vi "Helper SubVI - Simulate ECG Signal.vi"() -> (3 "Data":dynamicdata(graph))   [LabVIEW 2023]
doc: "Simulates an ECG signal."
uses:
  Instance           3 30Saved   subSimulate ECG Signal .vi
  <vilib>/measure/NI_MABase.lvlib
  <vilib>/Analysis/NI_AALBase.lvlib
panel:
  in  "Simulate Acquisition Timing?":bool=TRUE
  in  "Amplitude":dbl=1.0 format="%0.2f"
  in  "Isoelectric Voltage":dbl format="%0.2f"
  out "error out":errorcluster
  in  "QRS-T Delay (ms)":dbl(slide)=22.0 scale=0.0..40.0
  in  "P-QRS Delay (ms)":dbl(slide)=22.0 scale=0.0..40.0
  in  "60 Hz Noise\nAmplitude":dbl(knob) scale=0.0..1.0
  in  "White Noise \nAmplitude":dbl(knob) scale=0.0..1.0
  in  "error in (no error)":errorcluster
  in  "Number of Samples":i32=500
  in  "BPM":dbl(knob)=80.0 scale=40.0..140.0
  in  "Signal Type":T1(ring)=enum."Normal (random)"
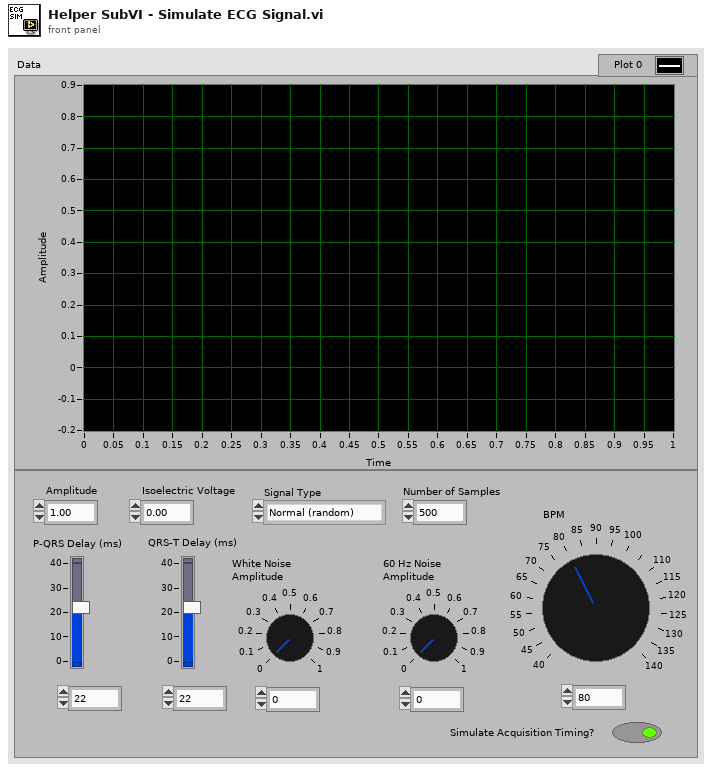
[diagram p1: front panel]
types:
  T1 = enum16{"Normal (regular)", "Normal (random)", "Hyperkalemia", "Atrial Tachycardia"}
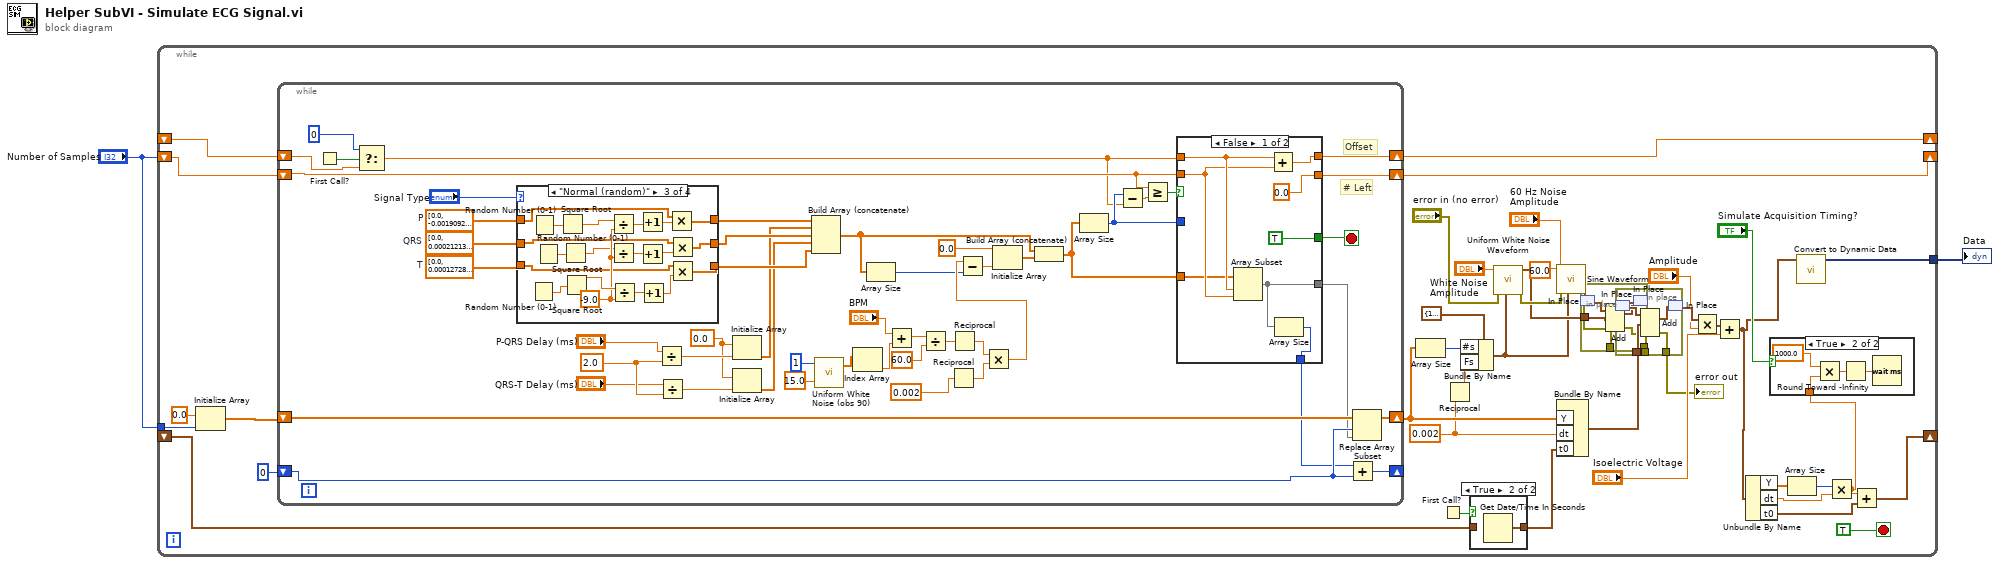
[diagram p0: block diagram]
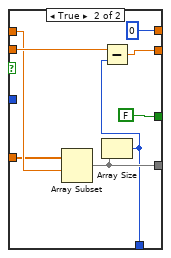
[diagram p4: hidden frame]
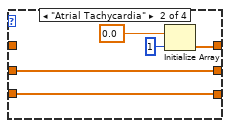
[diagram p6: hidden frame]
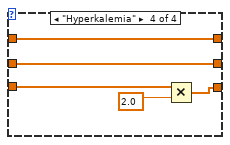
[diagram p7: hidden frame]
diagram:
  n1 = while {
    shift-right: [w6] -> _
    shift-left: _ -> [w36]
    shift-right: [w45] -> _
    shift-left: _ -> [w43]
    shift-right: [w44] -> _
    shift-left: "Number of Samples" -> [w42]
    tunnel: "Number of Samples" -> [w35]
    tunnel: [w3] -> w1
    stop <- TRUE stop-if-true
    w22 = 0.002 ("dt")
    n2 = Initialize Array(0.0 ("element"), w35) -> (w39:dbl[])
    n3 = while {
      shift-right: [w83] -> w45
      shift-left: w43 -> [w89]
      shift-right: [w82] -> w44
      shift-left: w42 -> [w86]
      shift-right: [w79] -> w26
      shift-left: w39 -> [w78]
      shift-right: [w77] -> _
      shift-left: 0 -> [w76]
      stop <- w87 stop-if-true
      w70 = dbl[] [0.0, 0.00012728044123886295, 0.0033092914722104368, 0.004963937208315655, 0.008909630886720407, 0.010691557064064489, 0.01463725074246924, 0.01641917691981332, 0.019601187950784894, 0.019983029274501487, 0.02189223589308443, 0.02609249045396691, 0.029529062367416203, 0.032965634280865505, 0.03703860840050912, 0.03945693678404752, 0.03971149766652524, 0.04174798472634705, 0.04645736105218498, 0.049130250318201105, 0.04951209164191769, 0.05167585914297836, 0.05434874840899448, 0.054730589732711075, 0.057403478998727185, 0.058930844293593555, 0.059439966058549, 0.060076368264743316, 0.061476453118370813, 0.0652948663555367, 0.068731438268986, 0.075222740772168, 0.08285956724649977, 0.08985999151463725, 0.09698769622401357, 0.10424268137462876, 0.11086126431904965, 0.11811624946966481, 0.1288078065337293, 0.1380992787441663, 0.14446330080610947, 0.15146372507424694, 0.16100975816716165, 0.17259227831989818, 0.18302927450148493, 0.18990241832838353, 0.1993211709800594, 0.20963088672040728, 0.21624946966482816, 0.22643190496393717, 0.2359779380568519, 0.2428510818837505, 0.25354263894781504, 0.26296139159949083, 0.2686890114552397, 0.27212558336868903, 0.2754348748408994, 0.27950784896054304, 0.28230801866779803, 0.28256257955027575, 0.28459906661009754, 0.28816291896478574, 0.287908358082308, 0.28408994484514216, 0.28243529910903686, 0.28230801866779803, 0.2783623249893933, 0.27785320322443785, 0.2763258379295715, 0.26843445057276194, 0.26092490453966904, 0.2543063215952482, 0.2466694951209164, 0.23635977938056854, 0.22210436996181587, 0.2092490453966907, 0.19881204921510393, 0.18442935935511243, 0.17221043699618158, 0.16126431904963937, 0.14662706830717012, 0.13478998727195587, 0.1247348324140857, 0.11391599490878235, 0.10322443784471785, 0.09278744166313109, 0.08184132371658889, 0.07102248621128554, 0.06313109885447603, 0.05651251591005515, 0.049130250318201105, 0.04162070428510819, 0.037165888841747985, 0.03322019516334323, 0.025710649130250316, 0.017946542214679676, 0.012728044123886296, 0.009418752651675858, 0.005473058973271107, 0.004963937208315655, 0.0040729741196436145, 0.0002545608824777259, -0.00038184132371658886, 0.00012728044123886295, 0.0]  # T
      w71 = dbl[] [0.0, 0.00021213406873143826, 0.00021213406873143826, -0.002545608824777259, -0.008273228680526093, -0.01675859142978362, -0.02821383114128129, -0.03988120492151039, -0.050912176495545185, -0.06257955027577429, -0.07721680101824353, -0.09291472210436996, -0.10797624098430209, -0.12091641917691981, -0.12558336868901146, -0.12006788290199406, -0.10670343657191345, -0.08994484514212983, -0.06618582944420874, -0.037335596096733134, -0.007212558336868901, 0.028638099278744167, 0.060670343657191345, 0.09079338141705558, 0.14064488756894358, 0.20767925328807807, 0.2931692829868477, 0.4007212558336869, 0.523759015697921, 0.6478574459058125, 0.756045820958846, 0.8332626219770896, 0.8699618158676283, 0.8606279168434451, 0.8039881204921511, 0.7019516334323292, 0.5717013152312261, 0.42426813746287656, 0.2675010606703437, 0.13131098854476028, -0.001484938481120068, -0.1175222740772168, -0.13003818413237167, -0.1130674586338566, -0.11221892235893084, -0.10521849809079338, -0.09652100127280441, -0.08124734832414086, -0.058124734832414086, -0.040729741196436145, -0.02821383114128129, -0.018667798048366567, -0.011879507848960543, -0.0067882901994060245, -0.0027577428935086977, 0.0]  # QRS
      w72 = dbl[] [0.0, -0.0019092066185829445, 0.0057276198557488335, 0.01972846839202376, 0.037759864234196014, 0.057064064488756894, 0.07106491302503182, 0.0831565549427238, 0.10182435299109037, 0.11349172677131947, 0.11561306745863385, 0.11540093338990241, 0.11731014000848536, 0.11073398387781078, 0.09821807382265592, 0.09270258803563852, 0.08336868901145524, 0.07042851081883751, 0.0587611370386084, 0.0460330929147221, 0.03797199830292745, 0.031607976240984305, 0.01951633432329232, 0.010182435299109036, 0.008061094611794654, 0.008273228680526093, 0.002333474756045821, -0.0008485362749257531, 0.00021213406873143826, 0.0]  # P
      w106 = 0.0 ("Element Data")
      w104 = 2.0 ("y")
      # "# Left"
      # "Offset"
      n4 = First Call?() -> (First Call?: T/F=w90:bool)
      n5 = Select(t=0, s=w90, f=w89) -> (s? t:f=w81:dbl)
      n6 = case shown="\"Normal (random)\"" "Signal Type" {
        tunnel: [w130 w133 w138 w156] -> w80
        tunnel: [w128 w131 w150 w159] -> w109
        tunnel: [w129 w132 w147 w157] -> w110
        tunnel: w72 -> [w130 _ w139 w156]
        tunnel: w71 -> [w129 w132 w137 w157]
        tunnel: w70 -> [w128 w131 w136 w155]
        frame "Normal (regular)", Default {
        }
        frame "Atrial Tachycardia" {
          n7 = Initialize Array(0.0 ("Element Data"), 1 ("Dimension Size")) -> (w133:dbl[])
        }
        frame "Normal (random)" {
          w148 = -9.0 ("y")
          n8 = Random Number (0-1)() -> (number: 0 to 1=w154:dbl)
          n9 = Random Number (0-1)() -> (number: 0 to 1=w143:dbl)
          n10 = Random Number (0-1)() -> (number: 0 to 1=w145:dbl)
          n11 = Square Root(x=w143) -> (sqrt(x)=w142:dbl)
          n12 = Square Root(x=w145) -> (sqrt(x)=w144:dbl)
          n13 = Square Root(x=w154) -> (sqrt(x)=w153:dbl)
          n14 = Divide(x=w142, y=w148) -> (x/y=w141:dbl)
          n15 = Divide(x=w144, y=w148) -> (x/y=w149:dbl)
          n16 = Divide(x=w153, y=w148) -> (x/y=w152:dbl)
          n17 = Increment(x=w141) -> (x+1=w140:dbl)
          n18 = Increment(x=w149) -> (x+1=w146:dbl)
          n19 = Increment(x=w152) -> (x+1=w151:dbl)
          n20 = Multiply(x=w139, y=w140) -> (x*y=w138:dbl[])
          n21 = Multiply(x=w137, y=w146) -> (x*y=w147:dbl[])
          n22 = Multiply(x=w136, y=w151) -> (x*y=w150:dbl[])
        }
        frame "Hyperkalemia" {
          n23 = Multiply(x=w155, y=2.0 ("Element Data")) -> (x*y=w159:dbl[])
        }
      }
      n24 = Divide(x="P-QRS Delay (ms)", y=w104) -> (x/y=w111:dbl)
      n25 = Divide(x="QRS-T Delay (ms)", y=w104) -> (x/y=w105:dbl)
      n26 = Initialize Array(w106, w111) -> (w108:dbl[])
      n27 = Initialize Array(w106, w105) -> (w107:dbl[])
      n28 = Build Array (concatenate)(w80, w108, w110, w107, w109) -> (w94:dbl[])
      n29 = call <vilib>:"Uniform White Noise (obs 90).vi"("amplitude"=15.0, "samples"=1) -> ("uniform white noise"=w65:dbl[])  [unwired: 1 in, 1 out]
      n30 = Index Array(array=w65) -> (element=w63:dbl)  [unwired: 1 in]
      n31 = Array Size(array=w94) -> (size(s)=w95:i32)
      n32 = Add(x="BPM", y=w63) -> (x+y=w62:dbl)
      n33 = Divide(x=w62, y=60.0) -> (x/y=w99:dbl)
      n34 = Reciprocal(x=0.002 ("dt")) -> (1/x=w100:dbl)
      n35 = Reciprocal(x=w99) -> (1/x=w98:dbl)
      n36 = Multiply(x=w98, y=w100) -> (x*y=w96:dbl)
      n37 = Subtract(x=w96, y=w95) -> (x-y=w97:dbl)
      n38 = Initialize Array(0.0 ("element"), w97) -> (w92:dbl[])
      n39 = Build Array (concatenate)(w94, w92) -> (w75:dbl[])
      n40 = Array Size(array=w75) -> (size(s)=w84:i32)
      n41 = Subtract(x=w84, y=w81) -> (x-y=w85:dbl)
      n42 = Greater Or Equal?(x=w86, y=w85) -> (x >= y?=w91:bool)
      n43 = case shown="False" w91 {
        tunnel: w81 -> [w116 w123]
        tunnel: w84 -> [_ _]
        tunnel: [TRUE FALSE] -> w87
        tunnel: w86 -> [w115 w125]
        tunnel: [w118 0 ("Number of Samples")] -> w83
        tunnel: [0.0 w124] -> w82
        tunnel: w75 -> [w114 w122]
        tunnel: [w112 w121] -> w74
        tunnel: [w113 w120] -> w73
        frame False {
          n44 = Array Subset(array=w114, index=w116, length=w115) -> (w112:dbl[])
          n45 = Add(x=w116, y=w115) -> (x+y=w118:dbl)
          n46 = Array Size(array=w112) -> (size(s)=w113:i32)
        }
        frame True {
          n47 = Array Subset(array=w122, index=w123) -> (w121:dbl[])  [unwired: 1 in]
          n48 = Array Size(array=w121) -> (size(s)=w120:i32)
          n49 = Subtract(x=w125, y=w120) -> (x-y=w124:dbl)
        }
      }
      n50 = Add(x=w73, y=w76) -> (x+y=w77:i32)
      n51 = Replace Array Subset(array=w78, new element=w74, index=w76) -> (w79:dbl[])
    }
    n52 = Array Size(array=w26) -> (size(s)=w23:i32)
    n53 = First Call?() -> (First Call?: T/F=w37:bool)
    n54 = Reciprocal(x=w22) -> (1/x=w21:dbl)
    n55 = Bundle By Name(cluster=cluster{"Fs":dbl, "#s":dbl} {"Fs"=1000.0, "#s"=1000.0} ("sampling info"), "#s"=w23, "Fs"=w21) -> (w24:cluster{"Fs":dbl, "#s":dbl})
    n56 = case shown="True" w37 {
      tunnel: [w60 w61] -> w34
      tunnel: w36 -> [w60 _]
      frame False {
      }
      frame True {
        n57 = Get Date/Time In Seconds() -> (seconds since 1Jan1904=w61:timestamp)
      }
    }
    n58 = call <vilib>:"Uniform White Noise Waveform.vi"("sampling info"=w24, "error in (no error)"="error in (no error)", "amplitude"="White Noise \nAmplitude") -> ("error out"=w33:errorcluster, "signal out"=w31:waveform(dbl))  [unwired: 2 in, 5 out]
    n59 = call <vilib>:"Sine Waveform.vi"("sampling info"=w24, "error in (no error)"=w33, "amplitude"="60 Hz Noise\nAmplitude", "frequency"=60.0) -> ("error out"=w27:errorcluster, "signal out"=w32:waveform(dbl))  [unwired: 3 in, 3 out]
    n60 = Bundle By Name("Y"=w26, "dt"=w22, "t0"=w34) -> (w28:waveform(dbl))  [unwired: 1 out]
    n61 = in-place {
      in-place-border: w31 -> [w49]
      in-place-border: [w47] -> w29
      in-place-border: w27 -> [w46]
      n62 = in-place-match #1(w32) -> (w50:waveform(dbl))
      n63 = Add(1:w49, 2:w50, 4:w46) -> (0:w48:waveform(dbl), 3:w47:errorcluster)
      n64 = in-place-match #1(w48) -> (w30:waveform(dbl))
    }
    n65 = in-place {
      in-place-border: w29 -> [w54]
      in-place-border: w28 -> [w53]
      in-place-border: [w51] -> w7
      n66 = in-place-match #2(w30) -> (w55:waveform(dbl))
      n67 = Add(1:w53, 2:w55, 4:w54) -> (0:w52:waveform(dbl), 3:w51:errorcluster)
      n68 = in-place-match #2(w52) -> (w15:waveform(dbl))
    }
    "error out" <- w7
    n69 = Multiply(x=w15, y="Amplitude") -> (x*y=w13:waveform(dbl))
    n70 = Add(x=w13, y="Isoelectric Voltage") -> (x+y=w4:waveform(dbl))
    n71 = Unbundle By Name(w4) -> ("Y"=w11:dbl[], "dt"=w9:dbl, "t0"=w8:timestamp)
    n72 = Array Size(array=w11) -> (size(s)=w10:i32)
    n73 = call "Convert to Dynamic Data"("Waveform"=w4) -> ("Dynamic Data Type"=w3:dynamicdata)  [unwired: 3 out]
    n74 = Multiply(x=w10, y=w9) -> (x*y=w5:dbl)
    n75 = case shown="True" "Simulate Acquisition Timing?" {
      tunnel: w5 -> [_ w58]
      frame False {
      }
      frame True {
        n76 = Multiply(x=1000.0 ("duration"), y=w58) -> (x*y=w57:dbl)
        n77 = Round Toward -Infinity(1:w57) -> (0:w56:dbl)
        n78 = Wait (ms)(milliseconds to wait=w56) -> ()  [unwired: 1 out]
      }
    }
    n79 = Add(x=w5, y=w8) -> (x+y=w6:timestamp)
  }
  "Data" <- w1
